vi "drive_straight4.vi"(5 "setpoint_hdg":dbl, 7 "setpoint_distance":dbl, 8 "reinit":bool, 9 "gyro_heading":dbl, 10 "vehspd_avg":dbl, 11 "distances":T1) -> (2 "done":bool, 3 "mpower":cluster{"left":dbl, "right":dbl})   [LabVIEW 2014]
panel:
  in  "max volt applied":dbl=1.0
  in  "drift_gain_backward":dbl=0.005
  out "drift const":dbl(graph)
  out "gyro":dbl(graph)
  in  "drift_gain_forward":dbl=0.005
  in  "vehspd_low_spd_lt":dbl=2.0
  in  "vehspd_lookup":dbl[](array[numeric])=[0.0, 1.0]
  in  "vehspd_prelookup":dbl[](array[numeric])=[0.0, 1.0]
  in  "rate_limit":dbl=1.0
  in  "distance gain":dbl=0.6
  in  "distance lead":dbl=1.0
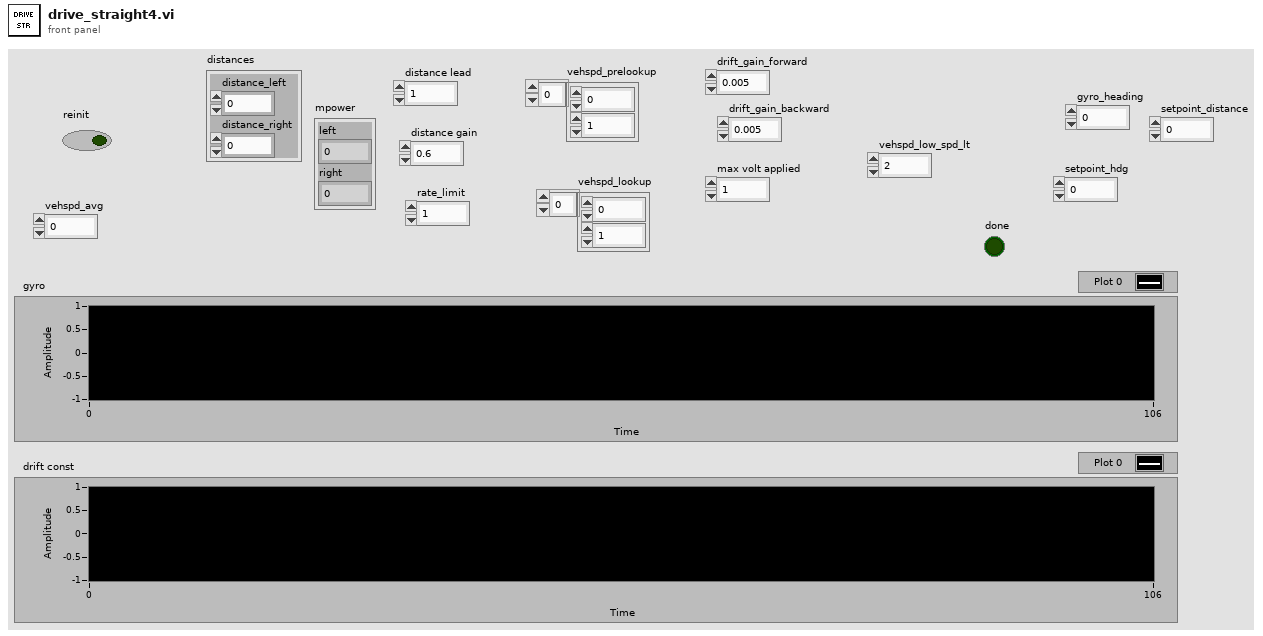
[diagram p1: front panel]
types:
  T1 = cluster{"distance_left":dbl, "distance_right":dbl}
  T2 = cluster{"setpoint_distance":dbl, "setpoint_distance":dbl}
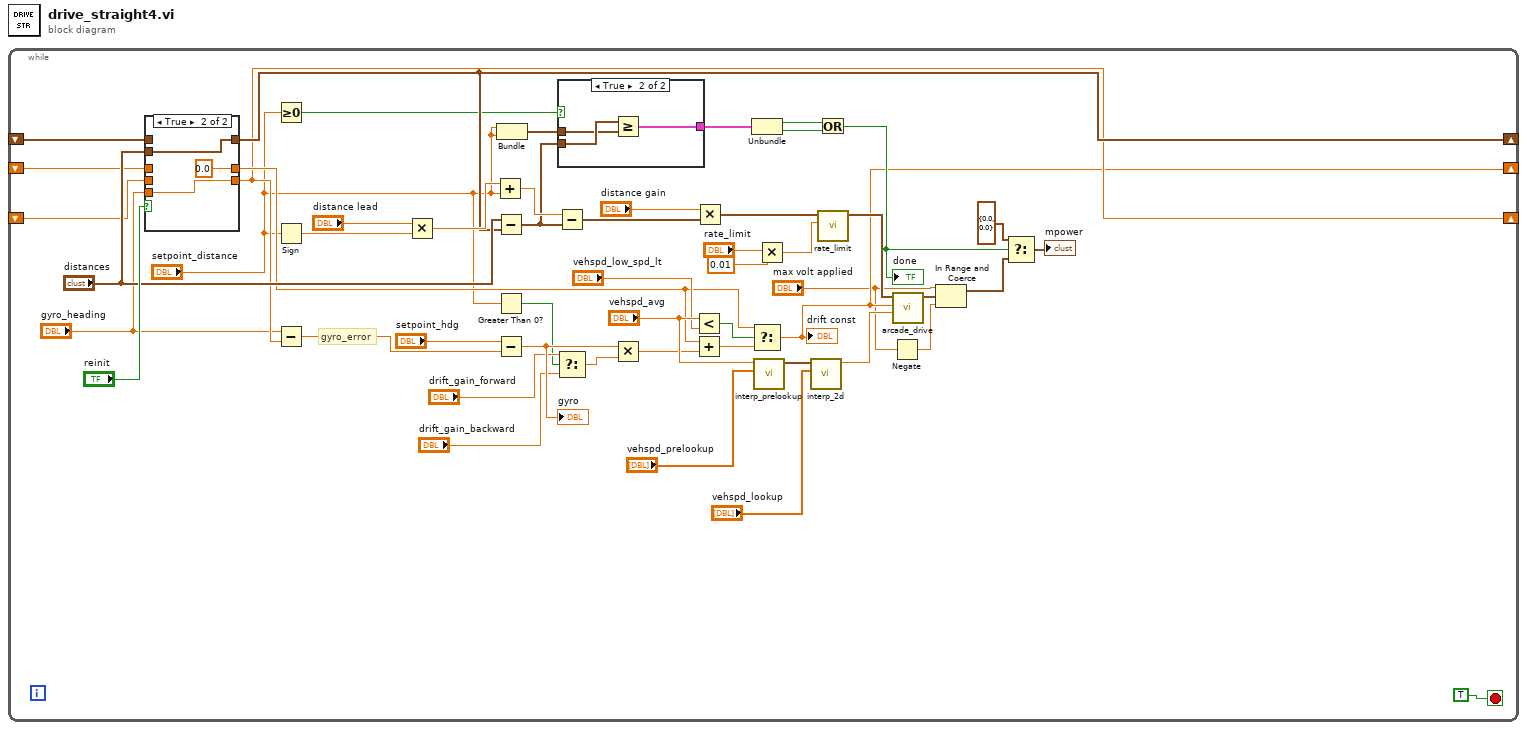
[diagram p0: block diagram]
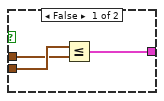
[diagram p2: hidden frame]
diagram:
  n1 = while {
    shift-right: [w44] -> _
    shift-left: _ -> [w50]
    shift-right: [w8] -> _
    shift-left: _ -> [w35]
    shift-right: [w21] -> _
    shift-left: _ -> [w22]
    stop <- TRUE stop-if-true
    # "gyro_error"
    n2 = case shown="True" "reinit" {
      tunnel: [w61 w64] -> w44
      tunnel: "distances" -> [_ w64]
      tunnel: w50 -> [w61 _]
      tunnel: [w60 0.0] -> w29
      tunnel: w35 -> [w60 _]
      tunnel: [w59 w62] -> w21
      tunnel: "gyro_heading" -> [_ w62]
      tunnel: w22 -> [w59 _]
      frame False {
      }
      frame True {
      }
    }
    n3 = Greater Or Equal To 0?(x="setpoint_distance") -> (x >= 0?=w28:bool)
    n4 = Sign(1:"setpoint_distance") -> (0:w48:dbl)
    n5 = Subtract(x="gyro_heading", y=w21) -> (x-y=w19:dbl)
    n6 = Multiply(x="distance lead", y=w48) -> (x*y=w47:dbl)
    n7 = Add(x=w47, y="setpoint_distance") -> (x+y=w46:dbl)
    n8 = Subtract(x="distances", y=w44) -> (x-y=w5:T1)
    n9 = Greater Than 0?(x="setpoint_distance") -> (x > 0?=w14:bool)
    n10 = Subtract(x="setpoint_hdg", y=w19) -> (x-y=w23:dbl)
    "gyro" <- w23
    n11 = Bundle("setpoint_distance"="setpoint_distance", "setpoint_distance"="setpoint_distance") -> (w4:T2)  [unwired: 1 in]
    n12 = Subtract(x=w46, y=w5) -> (x-y=w43:T1)
    n13 = Select(t="drift_gain_forward", s=w14, f="drift_gain_backward") -> (s? t:f=w16:dbl)
    n14 = case shown="True" w28 {
      tunnel: w5 -> [w55 w58]
      tunnel: w4 -> [w54 w57]
      tunnel: [w53 w56] -> w25
      frame False {
        n15 = Less Or Equal?(x=w55, y=w54) -> (x <= y?=w53:cluster{bool, bool})
      }
      frame True {
        n16 = Greater Or Equal?(x=w58, y=w57) -> (x >= y?=w56:cluster{bool, bool})
      }
    }
    n17 = Multiply(x=w23, y=w16) -> (x*y=w18:dbl)
    n18 = Less?(x="vehspd_avg", y="vehspd_low_spd_lt") -> (x < y?=w32:bool)
    n19 = Add(x=w29, y=w18) -> (x+y=w24:dbl)
    n20 = Multiply(x="distance gain", y=w43) -> (x*y=w41:T1)
    n21 = Unbundle(w25) -> (w27:bool, w26:bool)
    n22 = Select(t=w29, s=w32, f=w24) -> (s? t:f=w8:dbl)
    "drift const" <- w8
    n23 = call "interp_prelookup.vi"("x"="vehspd_prelookup", "X"="vehspd_avg") -> ("prelookup"=w37:cluster{"frac":dbl, "num":u8})  [unwired: 8 in, 1 out]
    n24 = Multiply(x="rate_limit", y=0.01) -> (x*y=w2:dbl)
    n25 = call "interp_2d.vi"("z"="vehspd_lookup", "prelookup"=w37) -> ("z"=w31:dbl)  [unwired: 9 in]
    n26 = Or(x=w27, y=w26) -> (x .or. y?=w10:bool)
    "done" <- w10
    n27 = call "rate_limit.vi"("Max Delta Per Iteration"=w2, "Drive"=w41) -> ("Output"=w39:cluster{"Left":dbl, "Right":dbl})  [unwired: 9 in]
    n28 = Negate(x="max volt applied") -> (-x=w7:dbl)
    n29 = call "arcade_drive.vi"("velocity_rat"=w31, "turn"=w8, "mpower"=w39) -> ("mpower"=w38:cluster{"left":dbl, "right":dbl})  [unwired: 8 in]
    n30 = In Range and Coerce(upper limit="max volt applied", x=w38, lower limit=w7) -> (coerced(x)=w12:cluster{"left":dbl, "right":dbl})  [unwired: 1 out]
    n31 = Select(t=cluster{"left":dbl, "right":dbl} {"left"=0.0, "right"=0.0}, s=w10, f=w12) -> (s? t:f=→"mpower":cluster{"left":dbl, "right":dbl})
  }
